vi "Set Path.vi"(0 "GMaps API in":refnum<class "GMaps API.lvclass">, 1 "Path":T1={"Color"="", "Weight"="", "Destination State"="", "Destination City"=" ", "Destination Street"="", "Origin State"="", "Origin City"=" ", "Origin Street"=""}, 5 "error in (no error)":errorcluster) -> (14 "GMaps API out":refnum<class "GMaps API.lvclass">, 19 "error out":errorcluster)   [LabVIEW 2016, in "GMaps API.lvclass"]
doc: "Sets a set of one or more locations connected by a path to overlay on the map image."
uses:
  GMaps API.lvclass
  Controls/Path.ctl
  GMaps API.lvclass/GMaps API.ctl
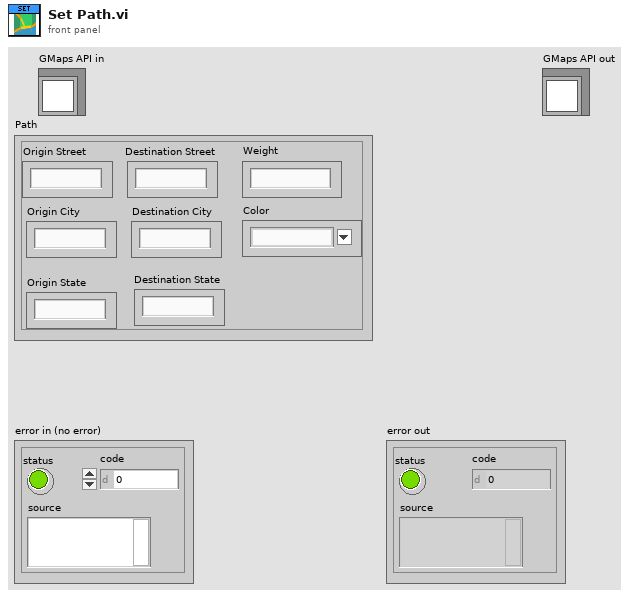
[diagram p1: front panel]
types:
  T1 = typedef "GMaps API.lvclass/Path.ctl" = cluster{"Color":string, "Weight":string, "Destination State":string, "Destination City":string, "Destination Street":string, "Origin State":string, "Origin City":string, "Origin Street":string}
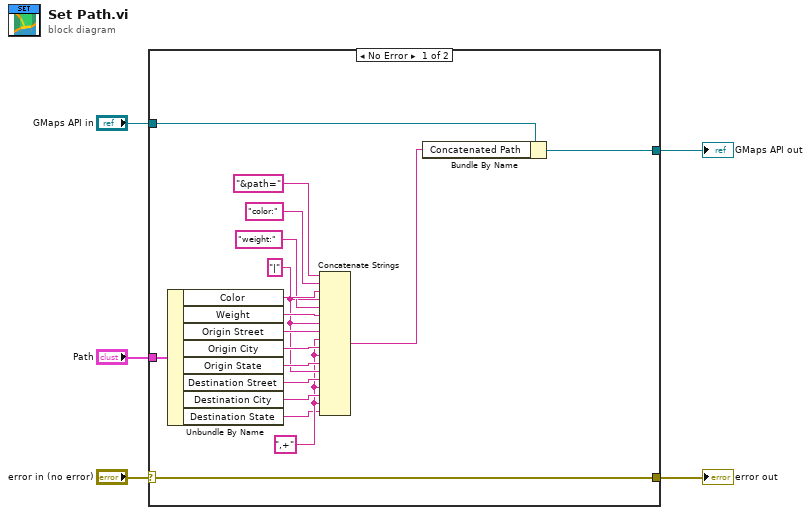
[diagram p0: block diagram]
diagram:
  n1 = case shown="No Error" "error in (no error)" {
    selector: "error in (no error)" -> [w23 w25]
    tunnel: [w23 w25] -> w4
    tunnel: [w19 w24] -> w3
    tunnel: "GMaps API in" -> [w22 w24]
    tunnel: "Path" -> [w21 _]
    frame No Error {
      w7 = ",+" ("string")
      w10 = "|"
      n2 = Unbundle By Name(w21) -> ("Color"=w16:string, "Weight"=w14:string, "Origin Street"=w13:string, "Origin City"=w12:string, "Origin State"=w11:string, "Destination Street"=w9:string, "Destination City"=w8:string, "Destination State"=w6:string)
      n3 = Concatenate Strings("&path=", "color:", w16, w10, "weight:", w14, w10, w13, w7, w12, w7, w11, w10, w9, w7, w8, w7, w6) -> (w20:string)
      n4 = Bundle By Name(cluster=w22, "Concatenated Path"=w20) -> (w19:refnum<class "GMaps API.lvclass">)
    }
    frame Error {
    }
  }
  "GMaps API out" <- w3
  "error out" <- w4
